vi "Get FPGA Setup Params.vi"(8 "error in (no error)":errorcluster, 10 "dummy":bool) -> (0 "error out":errorcluster, 1 "timed out?":bool, 2 "Reply Payload":T1={"Version String"="", "FPGA Setup Parameters"={"FPGA Timing Constraints"={"frame.length Min"=530, "frame.ST_OFF Min"=15, "frame.ST_ON Min"=8, "frame.first data idx"=14, "frame.integ Offset"=6, "frame.integ Delay"=3, "frame.ad_latch Delay"=11, "frame.trig time Max"=0}, "FPGA Timing Ctrl"={"trig.time"=220, "integ.count 1"=400, "integ.count 2"=350, "encdr.latch ctrl"=1, "pixel.read count"=512, "clock.select"=2, "ad.clock offset"=16, "data.control reg"=2}, "FPGA Laser Config"={"laser.gain"=10, "laser.threshold Low"=1400, "laser.threshold High"=1900, "laser.dac init"=912, "laser.dac Min"=800, "laser.dac Max"=4000, "laser.config reg"=3}, "FPGA Peak Proc Cfg"={"PD.threshold"=0, "PD.width detect Min"=0, "PD.sensor pixels"=512, "PD.config reg"=23}, "FPGA SPI Cfg"={"SPI Divide Value"=1, "SPI config reg"=1}}} {"FPGA Setup Parameters"."FPGA SPI Cfg"."SPI config reg" format="%03b"; "FPGA Setup Parameters"."FPGA Peak Proc Cfg"."PD.config reg" format="%05b"; "FPGA Setup Parameters"."FPGA Laser Config"."laser.config reg" format="%02b"; "FPGA Setup Parameters"."FPGA Timing Ctrl"."data.control reg" format="%03b"; "FPGA Setup Parameters"."FPGA Timing Constraints"."frame.trig time Max" format="%0.0f"})   [LabVIEW 2015, in "Tool Module.lvlib"]
doc: "Get the FPGA setup params that are saved in the Tool Module ToolModGLOB.vi. These were read from the Tool on startup.\n_____\nCreated using Delacor QMH Event Scripter 2.1.0.3.\n\n<b>Note:</b> This VI was modified by the <b>Validate DQMH Module</b> tool to turn off automatic error handling."
uses:
  Tool Module.lvlib
  Get FPGA Setup Params (Reply Payload)--cluster.ctl
  Tool Typedefs/_FPGA Setup Params Cluster--typedef.ctl
  Tool Typedefs/_FPGA Timing Constraints Cluster--typedef.ctl
  Tool Typedefs/_FPGA Timing Ctrl Cluster--typedef.ctl
  Tool Typedefs/_FPGA Laser Config Cluster--typedef.ctl
  Tool Typedefs/_FPGA Peak Proc Cfg Cluster--typedef.ctl
  Tool Typedefs/_FPGA SPI Cfg Cluster--typedef.ctl
  Get FPGA Setup Params Argument--cluster.ctl
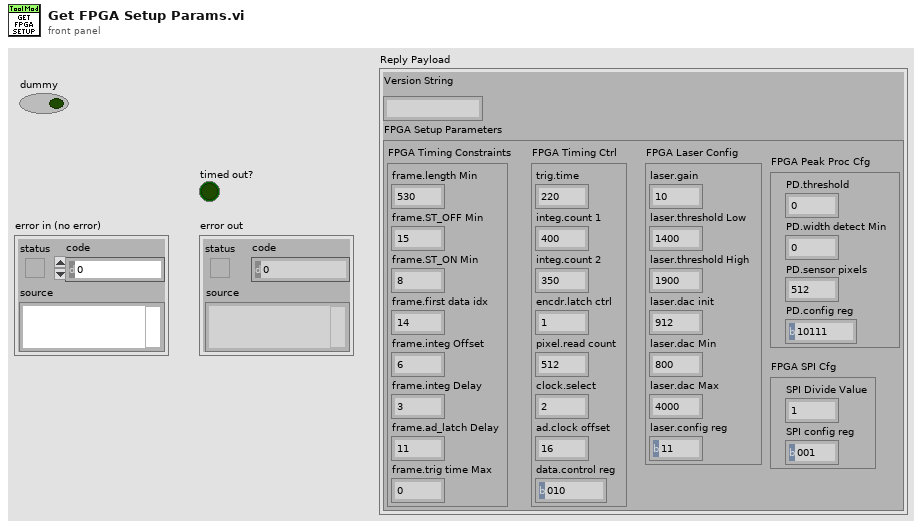
[diagram p1: front panel]
types:
  T1 = typedef "Tool Module.lvlib/Get FPGA Setup Params (Reply Payload)--cluster.ctl" = cluster{"Version String":string, "FPGA Setup Parameters":T2}
  T2 = typedef "_FPGA Setup Params Cluster--typedef.ctl" = cluster{"FPGA Timing Constraints":T3, "FPGA Timing Ctrl":T4, "FPGA Laser Config":T5, "FPGA Peak Proc Cfg":T6, "FPGA SPI Cfg":T7}
  T3 = typedef "_FPGA Timing Constraints Cluster--typedef.ctl" = cluster{"frame.length Min":u16, "frame.ST_OFF Min":u16, "frame.ST_ON Min":u16, "frame.first data idx":u16, "frame.integ Offset":u16, "frame.integ Delay":u16, "frame.ad_latch Delay":u16, "frame.trig time Max":u32}
  T4 = typedef "_FPGA Timing Ctrl Cluster--typedef.ctl" = cluster{"trig.time":u32, "integ.count 1":u32, "integ.count 2":u32, "encdr.latch ctrl":u32, "pixel.read count":u16, "clock.select":u16, "ad.clock offset":u16, "data.control reg":u16}
  T5 = typedef "_FPGA Laser Config Cluster--typedef.ctl" = cluster{"laser.gain":i16, "laser.threshold Low":u16, "laser.threshold High":u16, "laser.dac init":u16, "laser.dac Min":u16, "laser.dac Max":u16, "laser.config reg":u16}
  T6 = typedef "_FPGA Peak Proc Cfg Cluster--typedef.ctl" = cluster{"PD.threshold":u16, "PD.width detect Min":u8, "PD.sensor pixels":u16, "PD.config reg":u16}
  T7 = typedef "_FPGA SPI Cfg Cluster--typedef.ctl" = cluster{"SPI Divide Value":u8, "SPI config reg":u16}
  T8 = typedef "Tool Module.lvlib/Get FPGA Setup Params Argument--cluster.ctl" = cluster{"dummy":bool, "Wait Notifier":refnum<notifier>}
  T9 = typedef "Tool Module.lvlib/Request Events--cluster.ctl" = cluster{"Stop Module":refnum<user-event>, "Show Panel":refnum<user-event>, "Hide Panel":refnum<user-event>, "Get Module Execution Status":refnum<user-event>, "Show Diagram":refnum<user-event>, "GOTO":refnum<user-event>, "CONNECT":refnum<user-event>, "Get All Inspect Data":refnum<user-event>, "Start Data Monitor":refnum<user-event>, "Get FPGA Setup Params":refnum<user-event>, "Set FPGA Setup Params":refnum<user-event>, "Commit Tool Config":refnum<user-event>, "Set Integration Count":refnum<user-event>, "Set Laser Params":refnum<user-event>, "Get Mtrl Ctrl Reg":refnum<user-event>, "Commit Ctrl Reg":refnum<user-event>, "Write to File":refnum<user-event>, "Read from File":refnum<user-event>, "Set Device Temp Thresholds":refnum<user-event>, "Get Cycle Count":refnum<user-event>, "Return FPGA Setup Data":refnum<user-event>, "Update FPGA Setup Data":refnum<user-event>, "Setup Timer":refnum<user-event>, "Tool Status Reader Cmd":refnum<user-event>, "Stop Helper Loops":refnum<user-event>, "Enable Receive Stream":refnum<user-event>, "Get-Set Inspection Limits":refnum<user-event>, "INSPECT":refnum<user-event>, "Set EventLog Ref":refnum<user-event>}
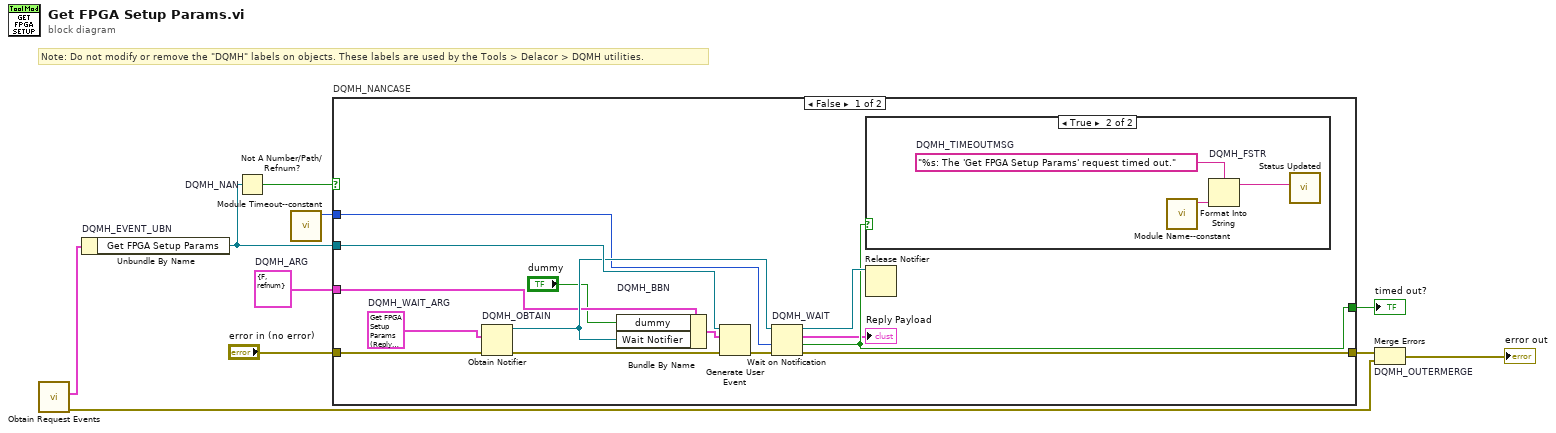
[diagram p0: block diagram]
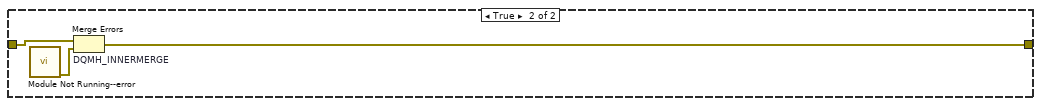
[diagram p3: hidden frame]
diagram:
  w4 = T8 {"dummy"=FALSE, "Wait Notifier"=refnum}  # DQMH_ARG
  # "Note: Do not modify or remove the \"DQMH\" labels on objects. These labels are used by the Tools > Delacor > DQMH utilities."
  n1 = call "Obtain Request Events.vi"() -> ("error out"=w2:errorcluster, "Tool Module Request Events"=w1:T9)  [unwired: 10 in]
  n2 = Unbundle By Name "DQMH_EVENT_UBN"(w1) -> ("Get FPGA Setup Params"=w8:refnum<user-event>)
  n3 = Not A Number/Path/Refnum? "DQMH_NAN"(number/path/refnum=w8) -> (NaN/Path/Refnum?=w7:bool)
  n4 = call "Module Timeout--constant.vi"() -> ("Module Timeout"=w3:i32)  [unwired: 11 in]
  n5 = case "DQMH_NANCASE" shown="False" w7 {
    tunnel: "error in (no error)" -> [w24 w30]
    tunnel: w8 -> [w22 _]
    tunnel: [w18 w29] -> w5
    tunnel: [w15 _] -> w6
    tunnel: w4 -> [w14 _]
    tunnel: w3 -> [w12 _]
    frame False {
      w19 = T1 {"Version String"="", "FPGA Setup Parameters"={"FPGA Timing Constraints"={"frame.length Min"=530, "frame.ST_OFF Min"=15, "frame.ST_ON Min"=8, "frame.first data idx"=14, "frame.integ Offset"=6, "frame.integ Delay"=3, "frame.ad_latch Delay"=11, "frame.trig time Max"=0}, "FPGA Timing Ctrl"={"trig.time"=220, "integ.count 1"=400, "integ.count 2"=350, "encdr.latch ctrl"=1, "pixel.read count"=512, "clock.select"=2, "ad.clock offset"=16, "data.control reg"=2}, "FPGA Laser Config"={"laser.gain"=10, "laser.threshold Low"=1400, "laser.threshold High"=1900, "laser.dac init"=912, "laser.dac Min"=800, "laser.dac Max"=4000, "laser.config reg"=3}, "FPGA Peak Proc Cfg"={"PD.threshold"=0, "PD.width detect Min"=0, "PD.sensor pixels"=512, "PD.config reg"=23}, "FPGA SPI Cfg"={"SPI Divide Value"=1, "SPI config reg"=1}}}  # DQMH_WAIT_ARG
      n6 = Obtain Notifier "DQMH_OBTAIN"(notification data type=w19, error in (no error)=w24) -> (notifier out=w17:refnum<notifier>, error out=w20:errorcluster)  [unwired: 2 in, 1 out]
      n7 = Bundle By Name "DQMH_BBN"(cluster=w14, "dummy"="dummy", "Wait Notifier"=w17) -> (w21:T8)
      n8 = Generate User Event(user event=w22, event data cluster=w21, error in=w20) -> (error out=w23:errorcluster)  [unwired: 1 in, 1 out]
      n9 = Wait on Notification "DQMH_WAIT"(notifier=w17, timeout in ms (-1)=w12, error in (no error)=w23) -> (notifier out=w16:refnum<notifier>, notification=→"Reply Payload":T1, timed out?=w15:bool, error out=w18:errorcluster)  [unwired: 1 in]
      n10 = case shown="True" w15 {
        frame False {
        }
        frame True {
          w27 = "%s: The 'Get FPGA Setup Params' request timed out."  # DQMH_TIMEOUTMSG
          n11 = call "Module Name--constant.vi"() -> ("Module Name"=w26:string)  [unwired: 11 in]
          n12 = Format Into String "DQMH_FSTR"(format string=w27, w26) -> (resulting string=w25:string)  [unwired: 2 in, 1 out]
          n13 = call "Status Updated.vi"("Status"=w25) -> ()  [unwired: 10 in, 1 out]
        }
      }
      n14 = Release Notifier(notifier=w16) -> ()  [unwired: 2 in, 3 out]
    }
    frame True {
      n15 = call "Module Not Running--error.vi"() -> ("error out"=w28:errorcluster)  [unwired: 11 in]
      n16 = Merge Errors "DQMH_INNERMERGE"(w30, w28) -> (w29:errorcluster)
    }
  }
  "timed out?" <- w6
  n17 = Merge Errors "DQMH_OUTERMERGE"(w5, w2) -> (→"error out":errorcluster)
